vi "Build Map--helper.vi"(10 "Measure":dbl[](array[numeric]), 11 "Array":string[](array[string])) -> (3 "Map":map{string, dbl}(c390))   [LabVIEW 2025, in "N4L_PSM3750_Interface.lvlib"]
uses:
  N4L_PSM3750_Interface.lvlib
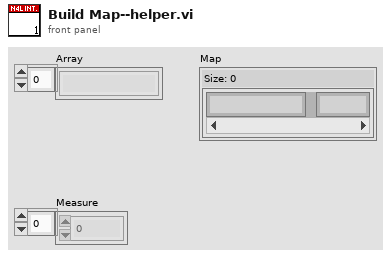
[diagram p1: front panel]
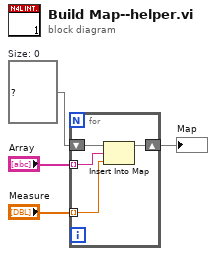
[diagram p0: block diagram]
diagram:
  w3 = map{string, dbl} {}  # Size: 0
  n1 = for {
    tunnel: "Measure" -> [w6] mode=indexing
    tunnel: "Array" -> [w5] mode=indexing
    shift-right: [w7] -> w4
    shift-left: w3 -> [w8]
    n2 = Insert Into Map(map in=w8, key=w5, value=w6) -> (map out=w7:map{string, dbl})  [unwired: 2 out]
  }
  "Map" <- w4
